vi "Stepper_plunger_Temp_Controller_23.vi"() -> ()   [LabVIEW 2018]
uses:
  <vilib>/Instr/_visa.llb/VISA Configure Serial Port (Instr).vi
  <vilib>/Waveform/WDTOps.llb/WDT Append Waveforms DBL.vi
panel:
  in  "Enum":T1(ring)
  in  "STOP Plunger":bool
  out "Temperature of Ethane 2":string
  out "Temperature of Ethane":waveform(dbl)(graph)
  in  "Stop for End of \nExperiment \nand Data Writing":bool
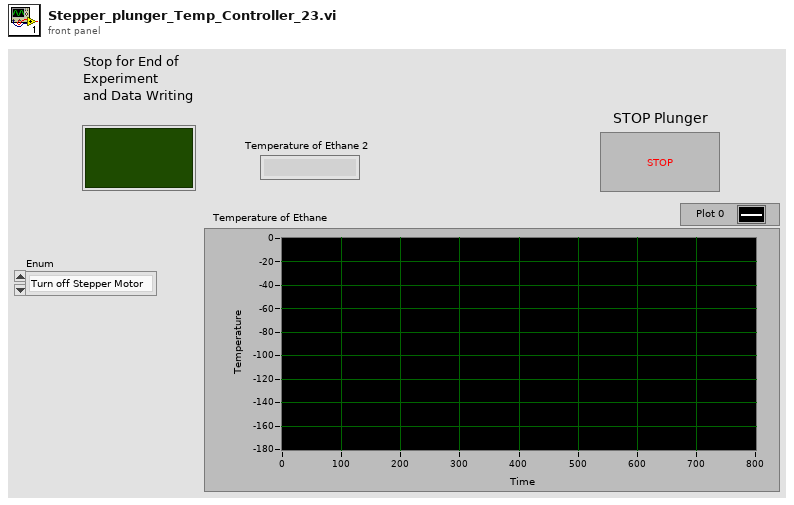
[diagram p1: front panel]
types:
  T1 = enum16{"Turn off Stepper Motor", "Turn  on Stepper Motor", "Move the Grid Down", "Move the Grid Up", "Stop the Grid Adjustment", "Start Plunging", "Reset Plunger", "Close Plunger Arm", "Open Plunger Arm"}
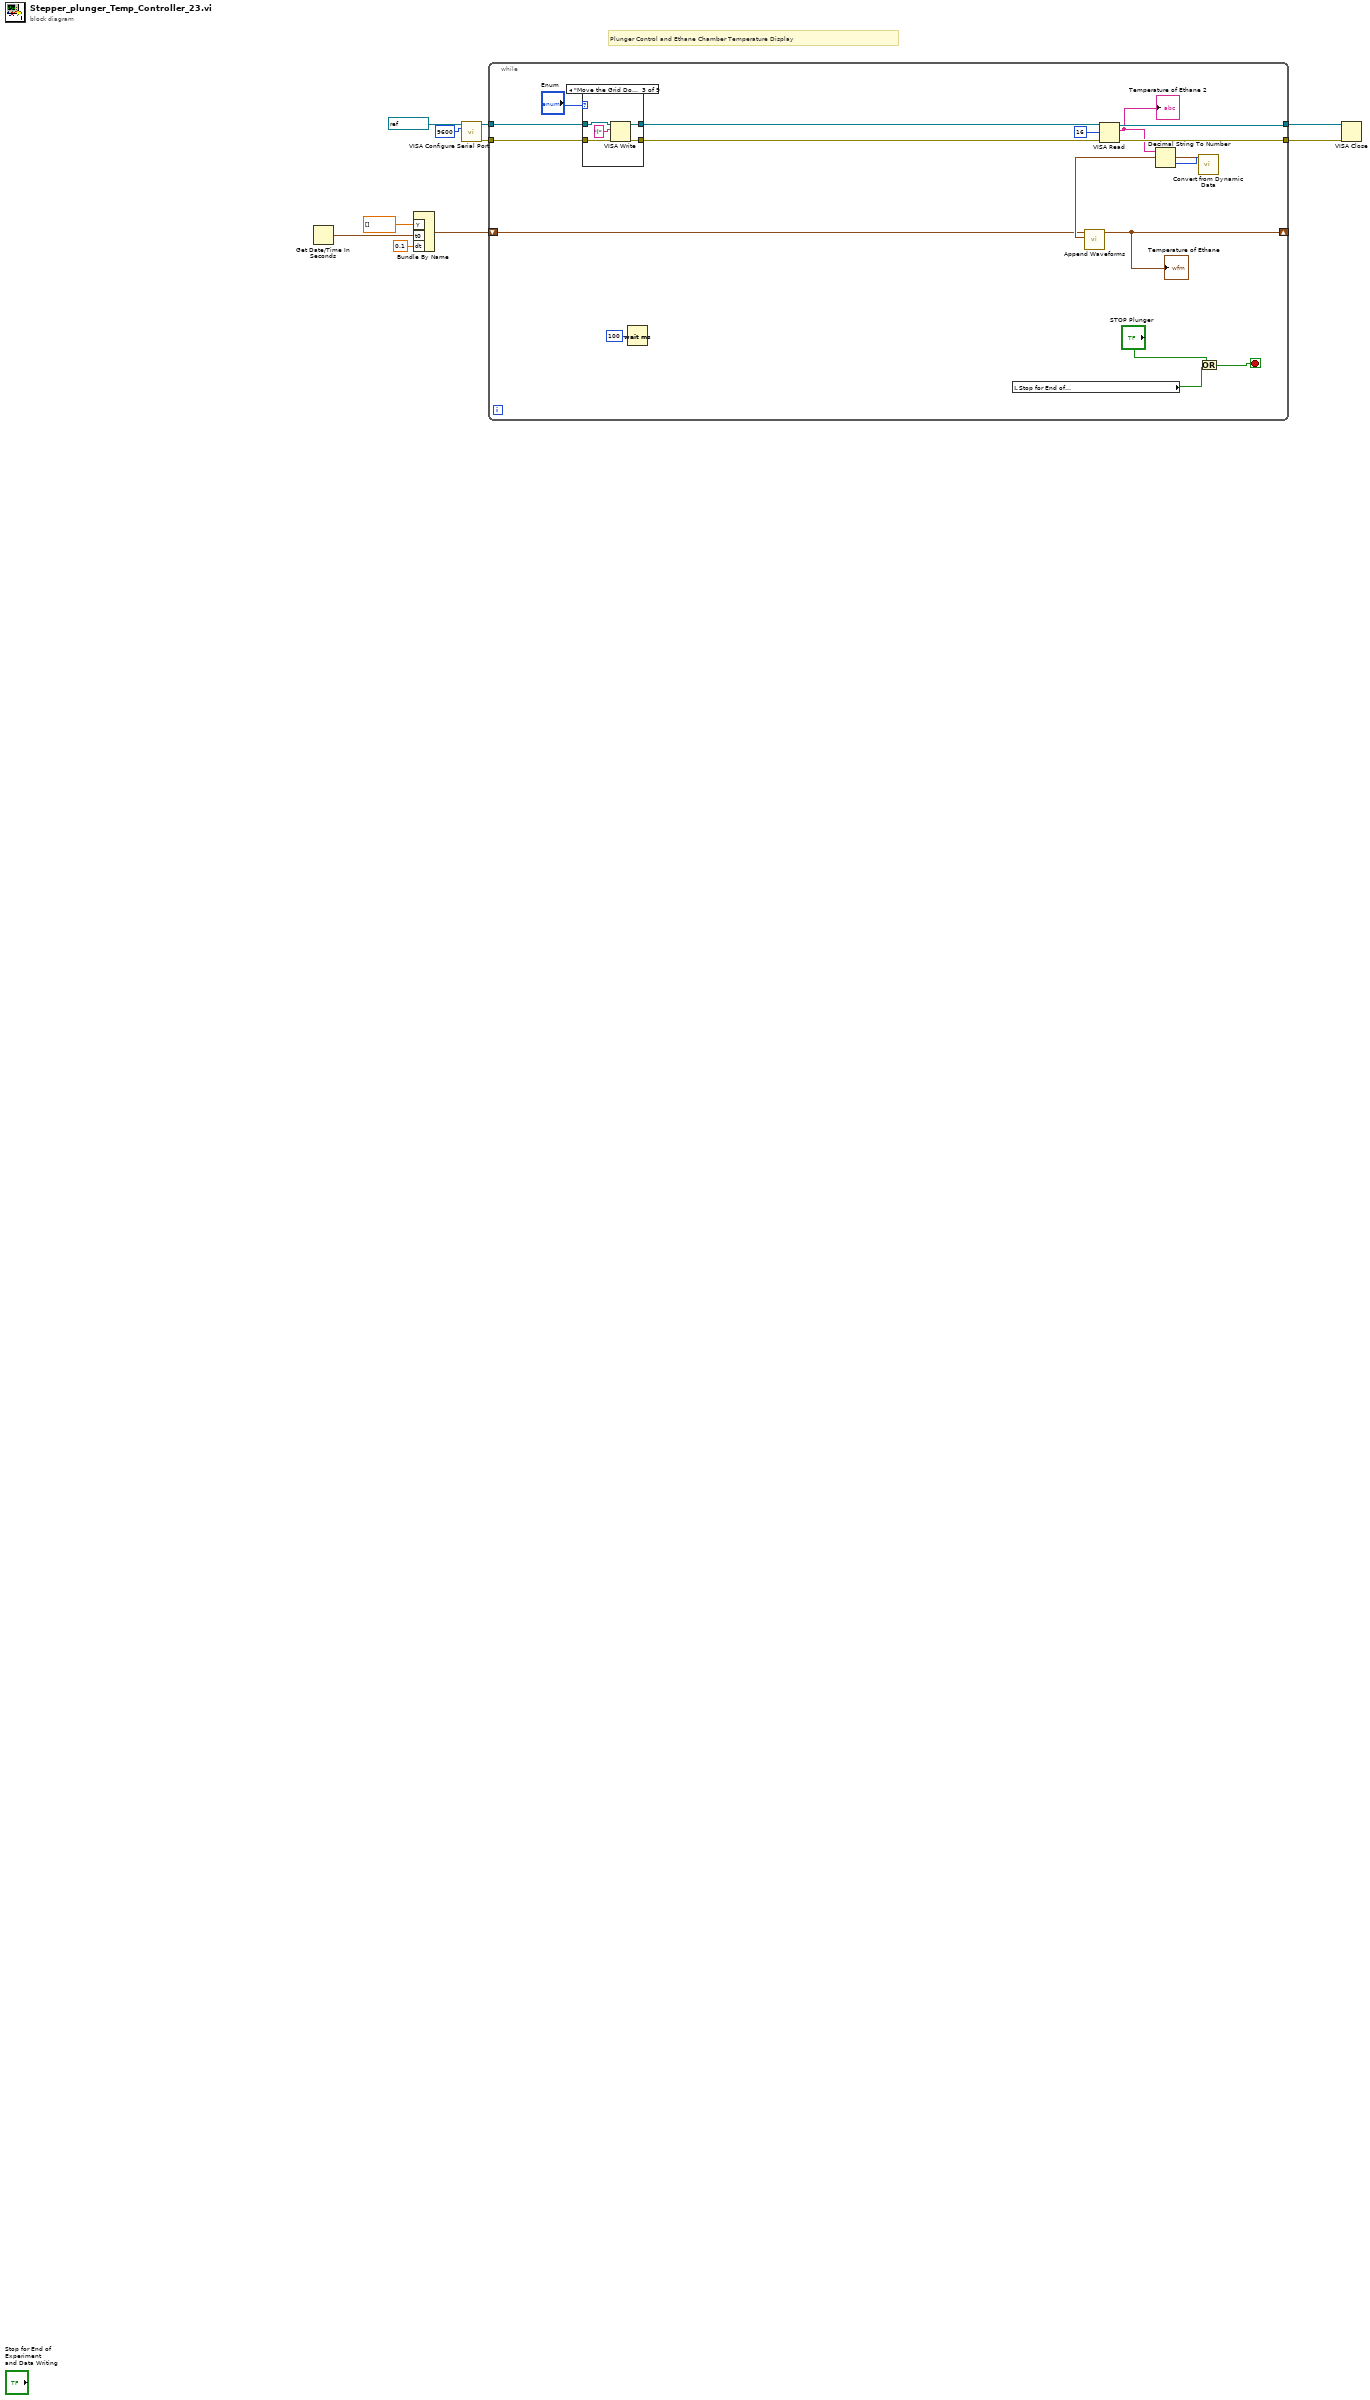
[diagram p0: block diagram]
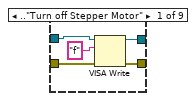
[diagram p2: hidden frame]
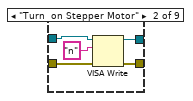
[diagram p3: hidden frame]
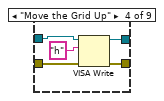
[diagram p4: hidden frame]
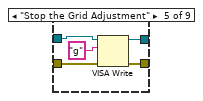
[diagram p5: hidden frame]
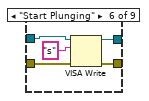
[diagram p6: hidden frame]
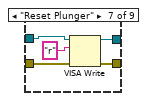
[diagram p7: hidden frame]
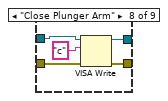
[diagram p8: hidden frame]
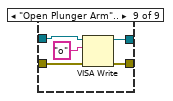
[diagram p9: hidden frame]
diagram:
  # "Plunger Control and Ethane Chamber Temperature Display"
  n1 = Get Date/Time In Seconds() -> (seconds since 1Jan1904=w3:timestamp)
  n2 = Bundle By Name("Y"=dbl[] [], "t0"=w3, "dt"=0.1) -> (w1:waveform(dbl))  [unwired: 1 in]
  n3 = call-poly "VISA Configure Serial Port"("VISA resource name"=refnum<visa-resource-name> "COM4", "baud rate (9600)"=u32 9600) -> ("VISA resource name out"=w8:refnum<visa-resource-name>, "error out"=w7:errorcluster)  [unwired: 12 in]
  n4 = while {
    tunnel: [w24] -> w10
    tunnel: [w23] -> w9
    tunnel: w8 -> [w27]
    tunnel: w7 -> [w26]
    shift-right: [w17] -> _
    shift-left: w1 -> [w18]
    stop <- w14 stop-if-true
    n5 = case shown="\"Move the Grid Down\"" "Enum" {
      tunnel: [w32 w37 w42 w47 w52 w57 w62 w67 w72] -> w13
      tunnel: [w31 w36 w41 w46 w51 w56 w61 w66 w71] -> w12
      tunnel: w27 -> [w30 w35 w40 w45 w50 w55 w60 w65 w70]
      tunnel: w26 -> [w29 w34 w39 w44 w49 w54 w59 w64 w69]
      frame .."Turn off Stepper Motor" {
        n6 = VISA Write(VISA resource name=w30, write buffer="f", error in (no error)=w29) -> (VISA resource name out=w32:refnum<visa-resource-name>, error out=w31:errorcluster)  [unwired: 1 out]
      }
      frame "Turn  on Stepper Motor" {
        n7 = VISA Write(VISA resource name=w35, write buffer="n", error in (no error)=w34) -> (VISA resource name out=w37:refnum<visa-resource-name>, error out=w36:errorcluster)  [unwired: 1 out]
      }
      frame "Move the Grid Down" {
        n8 = VISA Write(VISA resource name=w40, write buffer="l", error in (no error)=w39) -> (VISA resource name out=w42:refnum<visa-resource-name>, error out=w41:errorcluster)  [unwired: 1 out]
      }
      frame "Move the Grid Up" {
        n9 = VISA Write(VISA resource name=w45, write buffer="h", error in (no error)=w44) -> (VISA resource name out=w47:refnum<visa-resource-name>, error out=w46:errorcluster)  [unwired: 1 out]
      }
      frame "Stop the Grid Adjustment" {
        n10 = VISA Write(VISA resource name=w50, write buffer="g", error in (no error)=w49) -> (VISA resource name out=w52:refnum<visa-resource-name>, error out=w51:errorcluster)  [unwired: 1 out]
      }
      frame "Start Plunging" {
        n11 = VISA Write(VISA resource name=w55, write buffer="s", error in (no error)=w54) -> (VISA resource name out=w57:refnum<visa-resource-name>, error out=w56:errorcluster)  [unwired: 1 out]
      }
      frame "Reset Plunger" {
        n12 = VISA Write(VISA resource name=w60, write buffer="r", error in (no error)=w59) -> (VISA resource name out=w62:refnum<visa-resource-name>, error out=w61:errorcluster)  [unwired: 1 out]
      }
      frame "Close Plunger Arm" {
        n13 = VISA Write(VISA resource name=w65, write buffer="c", error in (no error)=w64) -> (VISA resource name out=w67:refnum<visa-resource-name>, error out=w66:errorcluster)  [unwired: 1 out]
      }
      frame "Open Plunger Arm".. {
        n14 = VISA Write(VISA resource name=w70, write buffer="o", error in (no error)=w69) -> (VISA resource name out=w72:refnum<visa-resource-name>, error out=w71:errorcluster)  [unwired: 1 out]
      }
    }
    n15 = Wait (ms)(milliseconds to wait=u32 100) -> ()  [unwired: 1 out]
    n16 = local read "Stop for End of \nExperiment \nand Data Writing"() -> (w16:bool)
    n17 = VISA Read(VISA resource name=w13, byte count=16, error in (no error)=w12) -> (VISA resource name out=w24:refnum<visa-resource-name>, read buffer=w21:string, error out=w23:errorcluster)  [unwired: 1 out]
    "Temperature of Ethane 2" <- w21
    n18 = Decimal String To Number(string=w21) -> (number=w20:i32)  [unwired: 2 in, 1 out]
    n19 = call "Convert from Dynamic Data"("Dynamic Data Type"=w20) -> ("Waveform"=w19:waveform(dbl))  [unwired: 3 in]
    n20 = call-poly <vilib>:"Append Waveforms.vi"("waveform B"=w19, "waveform A"=w18) -> ("waveform out"=w17:waveform(dbl))  [unwired: 8 in, 1 out]
    "Temperature of Ethane" <- w17
    n21 = Or(x="STOP Plunger", y=w16) -> (x .or. y?=w14:bool)
  }
  n22 = VISA Close(VISA resource name=w10, error in (no error)=w9) -> ()  [unwired: 1 out]
